vi "Test Remove Test from Suite.vi"(8 "error in (no error)":errorcluster, 11 "LUnit Test Suite Tests in":refnum<class "LUnit Test Suite Tests.lvclass">) -> (0 "error out":errorcluster, 3 "LUnit Test Suite Tests out":refnum<class "LUnit Test Suite Tests.lvclass">)   [LabVIEW 2020, in "LUnit Test Suite Tests.lvclass"]
uses:
  LUnit Test Suite Tests.lvclass
  LUnit Test Suite Tests.lvclass/LUnit Test Suite Tests.ctl
  source/LUnit Test Case.lvclass
  Test Doubles/Test Case Test Double/Test Case Test Double.lvclass
  Test Doubles/Test Case Test Double/Methods.ctl
  source/LUnit Test Suite.lvclass
  <vilib>/Astemes/LUnit/Test Case.lvclass
panel:
  out "List of Runnables":string[](array[string])
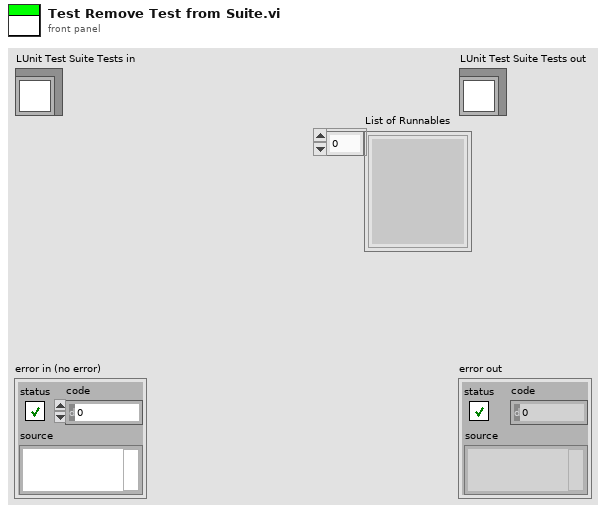
[diagram p1: front panel]
types:
  T1 = typedef "Test Case Test Double.lvclass/Methods.ctl" = enum16{"Test Failing Test.vi", "Test Passing Test.vi", "Test Error Test.vi", "Test Skip Test.vi", "Test Passing Pass If Test.vi", "Test Failing Pass If Test.vi", "Test Failing Fail If Test.vi", "Test Passing Fail If Test.vi", "Test Passing Pass If Error Test.vi", "Test Failing Pass If Error Test.vi", "Test Passing Fail If Error Test.vi", "Test Failing Fail If Error Test.vi", "Test Passing Pass If Equal Test.vi", "Test Failing Pass If Equal Test.vi", "Test Failing Fail If Equal Test.vi", "Test Passing Fail If Equal Test.vi", "Freezing Test.vi", "Test Pass on Expected Error Code.vi", "Test Error on Unexpected Error Code.vi", "Test Fail on Expected Error Code.vi", "Test Error when Fail on Unexpected Error Code.vi", "Test Pass on Expected Element in Array.vi", "Test Fail on Expected Element Not in Array.vi", "Test Pass on Expected Element in Set.vi", "Test Fail on Expected Element Not in Set.vi", "Test Pass on Expected Element in Map.vi", "Test Fail on Expected Element Not in Map.vi", "Test Fail on Unexpected Element in Array.vi", "Test Pass on Unexpected Element Not in Array.vi", "Test Fail if Unexpected Element in Set.vi", "Test Pass if Unexpected Element Not in Set.vi", "Test Fail if Unexpected Element in Map.vi", "Test Pass if Unexpected Element Not in Map.vi", "Test Pass on Expected Element in Array of Clusters.vi", "Test Pass on Expected Element Not in Array of Clusters.vi", "Test Matching String Test.vi", "Test Not Matching String Test.vi", "Verify Passing.vi", "Without Prefix.vi", "Private VI.vi"}
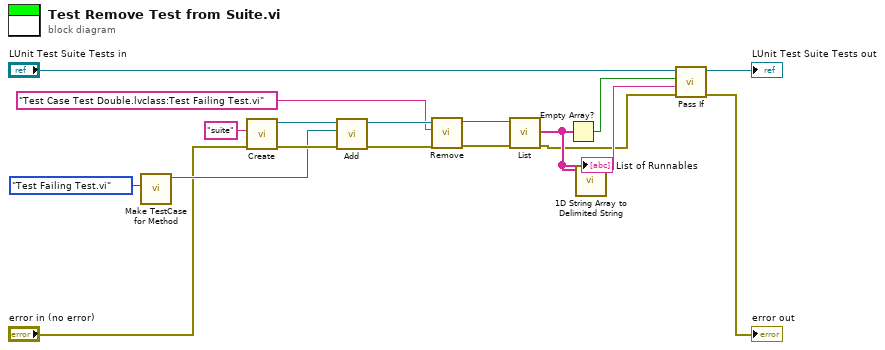
[diagram p0: block diagram]
diagram:
  n1 = call "Make TestCase for Method.vi"("Test Method"=Methods."Test Failing Test.vi") -> ("LUnit Test Case V2 out"=w14:refnum<class "LUnit Test Case.lvclass">)  [unwired: 9 in, 1 out]
  n2 = call "Create.vi"("error in (no error)"="error in (no error)", "Suite Name"="suite") -> ("error out"=w15:errorcluster, "LUnit Test Suite Out"=w16:refnum<class "LUnit Test Suite.lvclass">)  [unwired: 8 in]
  n3 = call "Add.vi"("error in (no error)"=w15, "Runnable"=w14, "LUnit Test Suite In"=w16) -> ("error out"=w11:errorcluster, "LUnit Test Suite Out"=w13:refnum<class "LUnit Test Suite.lvclass">)  [unwired: 7 in]
  n4 = call "Remove.vi"("error in (no error)"=w11, "Test to Remove"="Test Case Test Double.lvclass:Test Failing Test.vi" ("Name"), "LUnit Test Suite In"=w13) -> ("error out"=w9:errorcluster, "LUnit Test Suite Out"=w10:refnum<class "LUnit Test Suite.lvclass">)  [unwired: 7 in]
  n5 = call "List.vi"("error in (no error)"=w9, "LUnit Test Suite In"=w10) -> ("error out"=w2:errorcluster, "List of Runnables"=w4:string[])  [unwired: 8 in]
  "List of Runnables" <- w4
  n6 = Empty Array?(array=w4) -> (empty?=w5:bool)
  n7 = call <vilib>:"1D String Array to Delimited String.vi"("string array"=w4) -> ("delimited string"=w3:string)  [unwired: 10 in]
  n8 = call <vilib>:"Pass If.vi"("error in (no error)"=w2, "Message"=w3, "Pass?"=w5, "LUnit Test Case In"="LUnit Test Suite Tests in") -> ("error out"=→"error out":errorcluster, "LUnit Test Case Out"=→"LUnit Test Suite Tests out":refnum<class "LUnit Test Suite Tests.lvclass">)  [unwired: 6 in]
